vi "Get gRPC ID.vi"(11 "OOP Server in":refnum<class "ctet_mux.lvclass">) -> (2 "gRPC ID":T1, 3 "OOP Server out":refnum<class "ctet_mux.lvclass">)   [LabVIEW 2019, in "ctet_mux.lvlib" / "ctet_mux.lvclass"]
uses:
  ctet_mux.lvclass
  gRPC lvSupport/Server API/typeDefs/grpcId.ctl
  ctet_mux.lvclass/ctet_mux.ctl
  gRPC lvSupport/gprc-lvsupport.lvlib
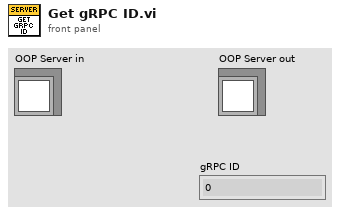
[diagram p1: front panel]
types:
  T1 = typedef "ctet_mux.lvlib/gprc-lvsupport.lvlib/grpcId.ctl" = u64
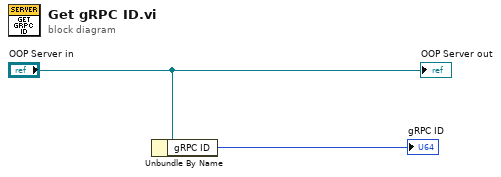
[diagram p0: block diagram]
diagram:
  n1 = Unbundle By Name("OOP Server in") -> ("gRPC ID"=→"gRPC ID":T1)
  "OOP Server out" <- "OOP Server in"
